vi "ReadKey(String).vi"(8 "error in":errorcluster, 9 "key":string, 10 "section":string, 11 "INIFileClass in":refnum<class "INIFileClass.lvclass">) -> (0 "error out":errorcluster, 2 "StringOut":string, 3 "INIFileClass out":refnum<class "INIFileClass.lvclass">)   [LabVIEW 2013, in "INIFileClass.lvclass"]
uses:
  INIFileClass.lvclass
  <vilib>/Utility/config.llb/Read Key (String).vi
  <vilib>/Utility/config.llb/NI_LVConfig.lvlib
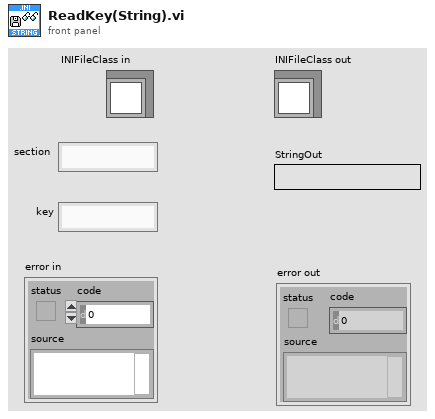
[diagram p1: front panel]
types:
  T1 = typedef "NI_LVConfig.lvlib/Config Data RefNum.ctl" = refnum<k1>
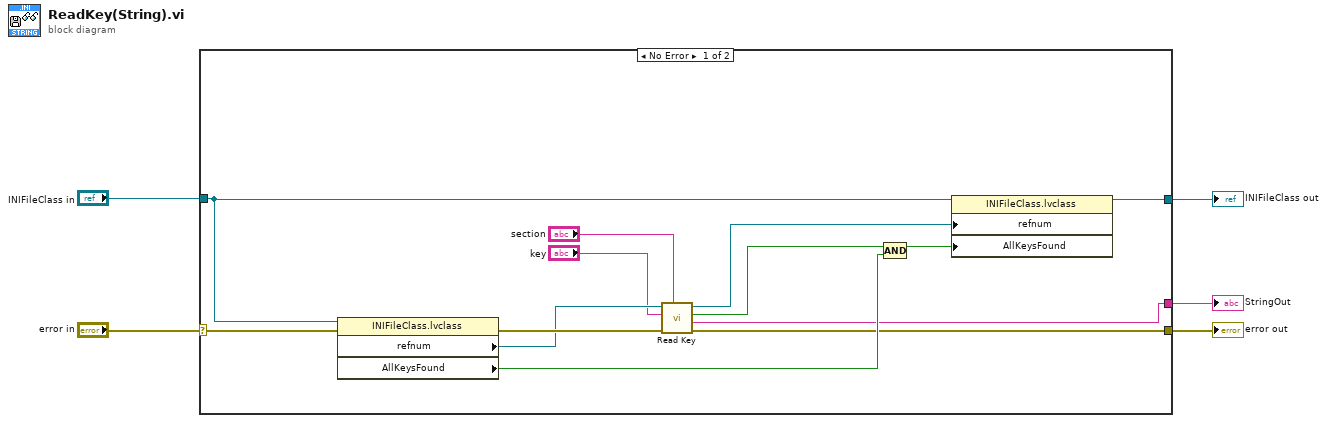
[diagram p0: block diagram]
diagram:
  n1 = case shown="No Error" "error in" {
    selector: "error in" -> [w12 w20]
    tunnel: [w11 w20] -> w4
    tunnel: [w8 w19] -> w2
    tunnel: "INIFileClass in" -> [w9 w19]
    tunnel: [w10 _] -> w1
    frame No Error {
      n2 = property class="INIFileClass.lvclass"(reference=w9, error in=w12) -> (error out=w18:errorcluster, "refnum"=w17:T1, "AllKeysFound"=w13:bool)  [unwired: 1 out]
      n3 = call-poly <vilib>:"Read Key.vi"("section"="section", "error in (no error)"=w18, "key"="key", "refnum"=w17) -> ("error out"=w11:errorcluster, "value"=w10:string, "found?"=w16:bool, "refnum out"=w15:T1)  [unwired: 4 in]
      n4 = Compound Arithmetic op=AND(w16, w13) -> (w14:bool)
      n5 = property class="INIFileClass.lvclass"(reference=w9, "refnum"=w15, "AllKeysFound"=w14) -> (reference out=w8:refnum<class "INIFileClass.lvclass">)  [unwired: 1 in, 1 out]
    }
    frame Error {
    }
  }
  "error out" <- w4
  "INIFileClass out" <- w2
  "StringOut" <- w1
